vi "ExeLogWrite.vi"(7 "Extra":string, 8 "refnum in":refnum<file>, 9 "State":string, 10 "Message":string, 11 "error in":errorcluster) -> (0 "refnum out":refnum<file>, 3 "error out":errorcluster)   [LabVIEW 2019]
uses:
  <vilib>/Utility/error.llb/DialogType.ctl
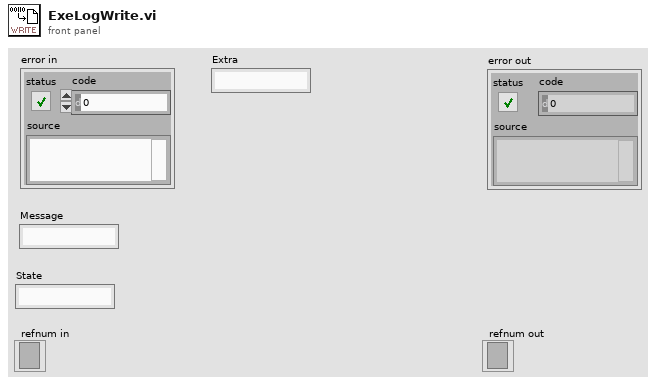
[diagram p1: front panel]
types:
  T1 = typedef "DialogType.ctl" = u16
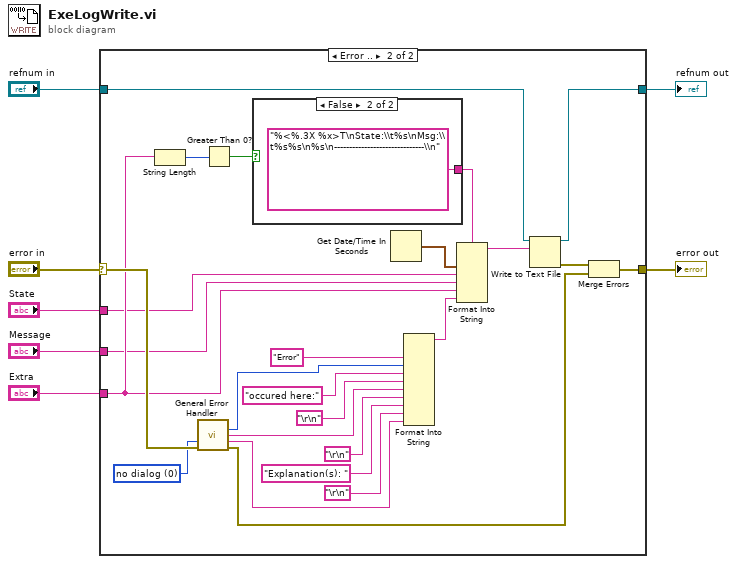
[diagram p0: block diagram]
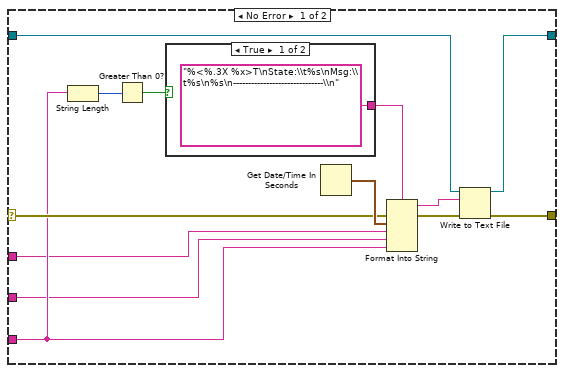
[diagram p2: hidden frame]
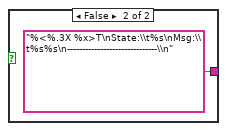
[diagram p3: hidden frame]
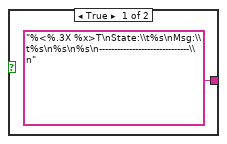
[diagram p4: hidden frame]
diagram:
  n1 = case shown="Error .." "error in" {
    selector: "error in" -> [w13 w35]
    tunnel: "refnum in" -> [w17 w37]
    tunnel: [w16 w36] -> w6
    tunnel: [w15 w32] -> w5
    tunnel: "Extra" -> [w10 w27]
    tunnel: "State" -> [w9 w24]
    tunnel: "Message" -> [w8 w25]
    frame No Error {
      n2 = String Length(string=w10) -> (length=w11:i32)
      n3 = Greater Than 0?(x=w11) -> (x > 0?=w12:bool)
      n4 = case shown="True" w12 {
        tunnel: ["%<%.3X %x>T\nState:\\t%s\nMsg:\\t%s\n%s\n------------------------------\\n" ("format string") "%<%.3X %x>T\nState:\\t%s\nMsg:\\t%s%s\n------------------------------\\n" ("format string")] -> w18
        frame True {
        }
        frame False {
        }
      }
      n5 = Get Date/Time In Seconds() -> (seconds since 1Jan1904=w19:timestamp)
      n6 = Format Into String(format string=w18, error in=w13, w19, w9, w8, w10) -> (resulting string=w20:string, error out=w14:errorcluster)  [unwired: 1 in]
      n7 = Write to Text File(file (use dialog)=w17, text=w20, error in=w14) -> (refnum out=w16:refnum<file>, error out=w15:errorcluster)  [unwired: 1 in, 1 out]
    }
    frame Error {
      w23 = T1 0 items=["no dialog", "OK message", "continue or stop message", "OK message + warnings", "continue/stop + warnings"] ("type of dialog (OK msg:1)")
      n8 = String Length(string=w27) -> (length=w28:i32)
      n9 = call <vilib>:"General Error Handler.vi"("type of dialog (OK msg:1)"=w23, "error in (no error)"=w35) -> ("code out"=w33:i32, "source out"=w44:string, "message"=w45:string, "error out"=w30:errorcluster)  [unwired: 9 in, 1 out]
      n10 = Greater Than 0?(x=w28) -> (x > 0?=w29:bool)
      n11 = case shown="False" w29 {
        tunnel: ["%<%.3X %x>T\nState:\\t%s\nMsg:\\t%s\n%s\n%s\n------------------------------\\n" ("format string") "%<%.3X %x>T\nState:\\t%s\nMsg:\\t%s%s\n%s\n------------------------------\\n" ("format string")] -> w26
        frame True {
        }
        frame False {
        }
      }
      n12 = Get Date/Time In Seconds() -> (seconds since 1Jan1904=w47:timestamp)
      n13 = Format Into String("Error", w33, "occured here:" ("input 3"), "\r\n", w44, "\r\n", "Explanation(s): ", "\r\n", w45) -> (resulting string=w34:string)  [unwired: 3 in, 1 out]
      n14 = Format Into String(format string=w26, w47, w24, w25, w27, w34) -> (resulting string=w46:string)  [unwired: 2 in, 1 out]
      n15 = Write to Text File(file (use dialog)=w37, text=w46) -> (refnum out=w36:refnum<file>, error out=w31:errorcluster)  [unwired: 2 in, 1 out]
      n16 = Merge Errors(w31, w30) -> (w32:errorcluster)
    }
  }
  "refnum out" <- w6
  "error out" <- w5
